vi "Get UserEvent.vi"(8 "error in":errorcluster, 11 "EventMessenger":refnum<class "EventMessenger.lvclass">) -> (0 "error out":errorcluster, 2 "Messenger Event":refnum<user-event>, 3 "EventMessenger out":refnum<class "EventMessenger.lvclass">)   [LabVIEW 2011, in "Messenging.lvlib" / "EventMessenger.lvclass"]
uses:
  EventMessenger.lvclass
  TextVarientMessage/MSG.lvclass
  EventMessenger.lvclass/EventMessenger.ctl
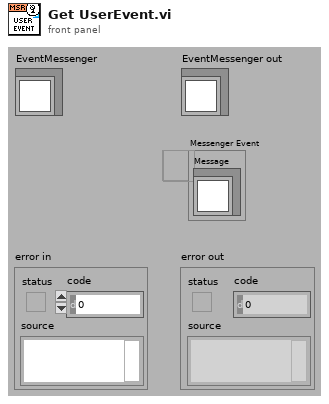
[diagram p1: front panel]
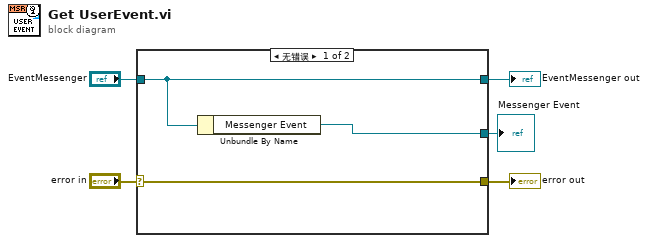
[diagram p0: block diagram]
diagram:
  n1 = case shown="无错误" "error in" {
    selector: "error in" -> [w7 w10]
    tunnel: [w7 w10] -> w4
    tunnel: [w8 w9] -> w2
    tunnel: "EventMessenger" -> [w8 w9]
    tunnel: [w6 _] -> w1
    frame No Error {
      n2 = Unbundle By Name(w8) -> ("Messenger Event"=w6:refnum<user-event>)
    }
    frame Error {
    }
  }
  "error out" <- w4
  "EventMessenger out" <- w2
  "Messenger Event" <- w1
